vi "Begin Str.vi"   [LabVIEW 2019, in "LabPack.lvlib" / "Reader.lvclass"]
doc: "Starts decoding a string. An error will occur if the current MessagePack object in the data is not a string."
uses:
  Reader.lvclass
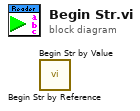
[diagram p0: block diagram]
diagram:
  n1 = call "Begin Str by Reference.vi"() -> ()  [unwired: 9 in, 3 out]
  n2 = call "Begin Str by Value.vi"() -> ()  [unwired: 9 in, 3 out]
